vi "getValue.vi"(8 "error in (no error)":errorcluster, 11 "XML Tree in":refnum<class "XML Tree.lvclass">) -> (0 "error out":errorcluster, 2 "Value":string, 3 "XML Tree out":refnum<class "XML Tree.lvclass">)   [LabVIEW 2013, in "XML Tree.lvclass"]
uses:
  XML Tree.lvclass
  XML Tree.lvclass/XML Tree.ctl
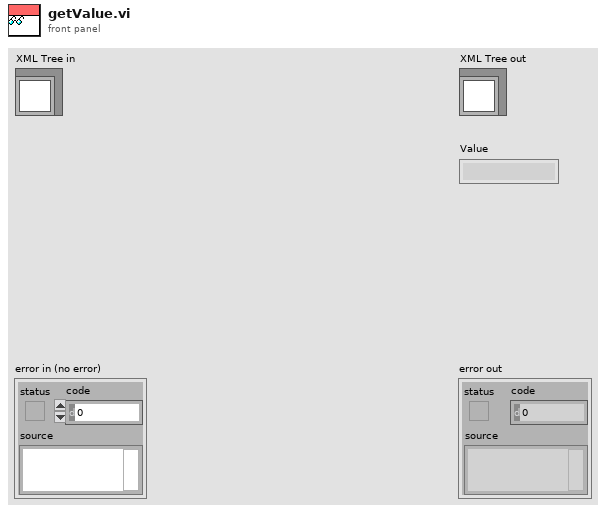
[diagram p1: front panel]
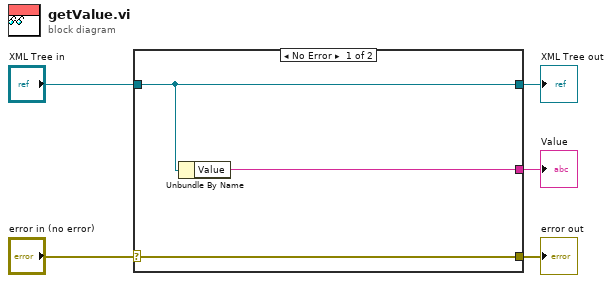
[diagram p0: block diagram]
diagram:
  n1 = case shown="No Error" "error in (no error)" {
    selector: "error in (no error)" -> [w8 w9]
    tunnel: [w8 w9] -> w4
    tunnel: [w7 w10] -> w2
    tunnel: "XML Tree in" -> [w7 w10]
    tunnel: [w6 _] -> w1
    frame No Error {
      n2 = Unbundle By Name(w7) -> ("Value"=w6:string)
    }
    frame Error {
    }
  }
  "error out" <- w4
  "XML Tree out" <- w2
  "Value" <- w1
